vi "Live TDMS Viewer.vi"() -> ()   [LabVIEW 2019, in "Report Viewer.lvlib" / "Report Viewer.lvclass"]
doc: "Defer all the request for panel update the panel list. This will improve the loading time."
uses:
  Report Viewer.lvclass
  Custom Controls/Browse Tools.ctl
  <vilib>/Utility/tdmsutil.llb/fileViewerConfigData.ctl
panel:
  in  "tdms file in":refnum<k34>
  in  "Display Format":T1(ring)
  in  "Settings":bool
  in  "Properties / Values / Graph":T2(tab)=enum."Analog values (graph)"
  in  "Properties":i32(listbox)
  in  "Raw data values":i32(listbox)=-1
  out "Delta X (Time mS)":dbl
  out "Delta Y (Amplitude)":dbl
  out "Waveform Graph":waveform(dbl)[](graph)=[{"t0"=timestamp(0 s since 1904-01-01), "dt"=1.0, "Y"=[]}]
  in  "File contents":string[](tree)=["\"\u0000\u0000\u0000\u0002\u0000\u0000\u0000+Halt Mode Running_11:25:18.755 AM 11/6/2019\u0000\u0000\u0000\nPJB1_S CH0\""]
  in  "Open TDMS":bool
  in  "Save Graph":bool
  in  "Save Data":bool
  in  "Finished":bool
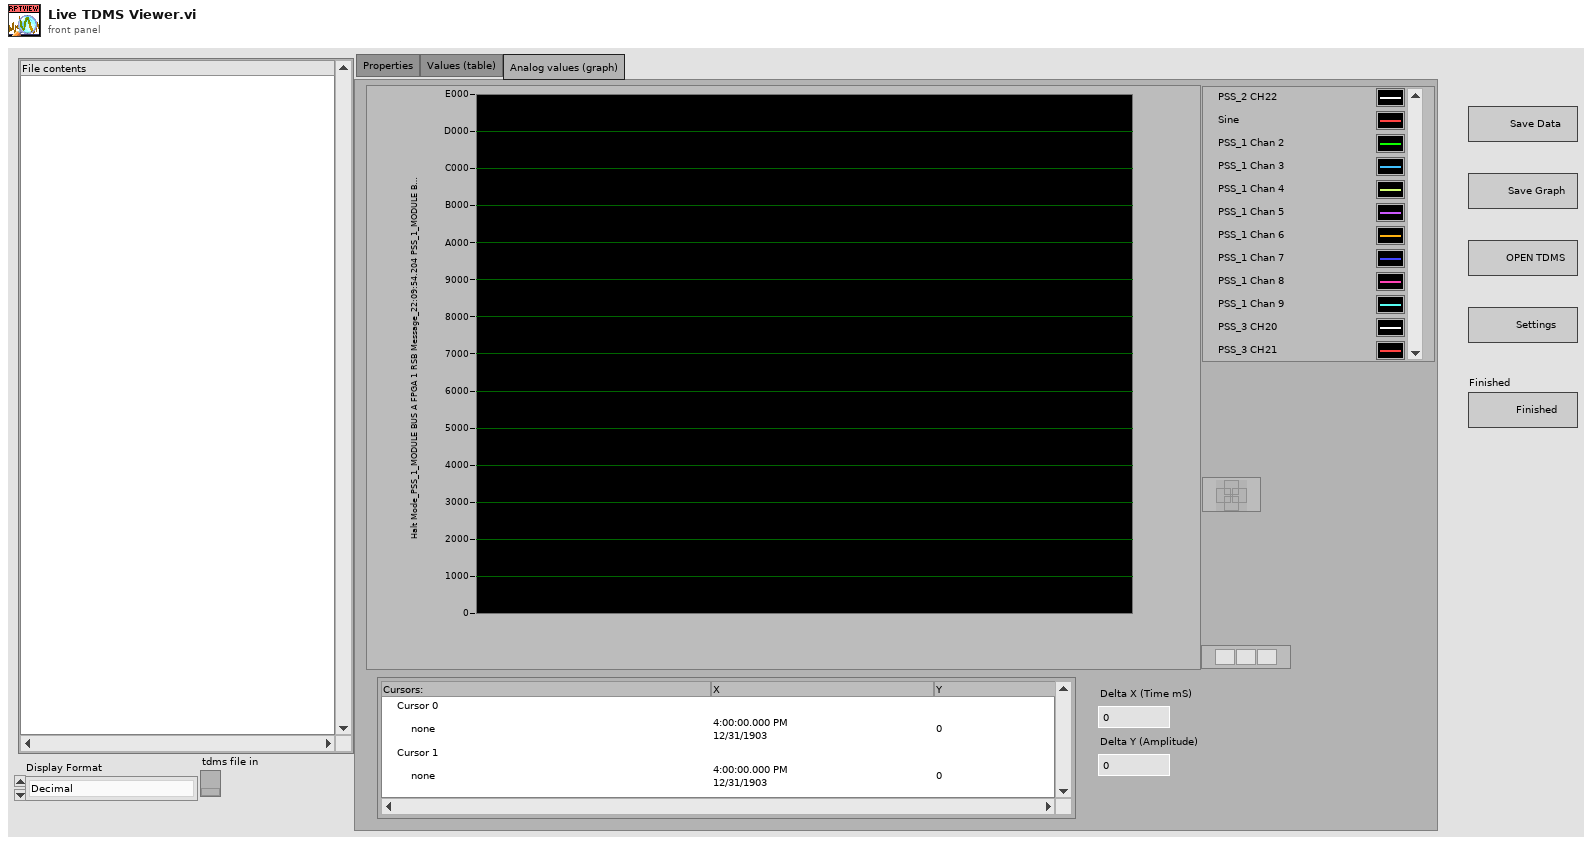
[diagram p1: front panel]
types:
  T1 = enum16{"Decimal", "Scientific", "Engineering", "Binary", "Octal", "Hexadecimal"}
  T2 = enum32{"Properties", "Values (table)", "Analog values (graph)"}
  T3 = typedef "fileViewerConfigData.ctl" = cluster{"Show all (table)":bool, "Show all (graph)":bool, "limit (table)":u64, "limit (graph)":u64, "no show":bool, "start (table)":u64, "start (graph)":u64}
  T4 = typedef "Report Viewer.lvlib/Report Viewer.lvclass/Browse Tools.ctl" = cluster{"Group":string, "Channel":string, "TDMS View Cfg":T3}
  T5 = typedef "imagedata.ctl" = cluster{"image type":i32, "image depth":i32, "image":u8[], "mask":u8[], "colors":u32[], "Rectangle":cluster{"left":i16, "top":i16, "right":i16, "bottom":i16}}
  T6 = typedef "LVCursorListTypeDef.ctl" = cluster{"Name":string, "Color":u32, "Style":u8, "Point Style":u8, "Name Visible":bool, "Allow Drag":bool, "Cursor Mode":u32, "Plot":i32, "Index":i32, "Position":cluster{"X":dbl, "Y":dbl}, "X Scale":u32, "Y Scale":u32, "Watch Plots":i32[], "Watch All Plots":bool, "Plot Area":i32, "Label Offset":cluster{"X":dbl, "Y":dbl}}[]
  T7 = cluster{"Name":string, "Color":u32, "Style":u8, "Point Style":u8, "Name Visible":bool, "Allow Drag":bool, "Cursor Mode":u32, "Plot":i32, "Index":i32, "Position":cluster{"X":dbl, "Y":dbl}, "X Scale":u32, "Y Scale":u32, "Watch Plots":i32[], "Watch All Plots":bool, "Plot Area":i32, "Label Offset":cluster{"X":dbl, "Y":dbl}}
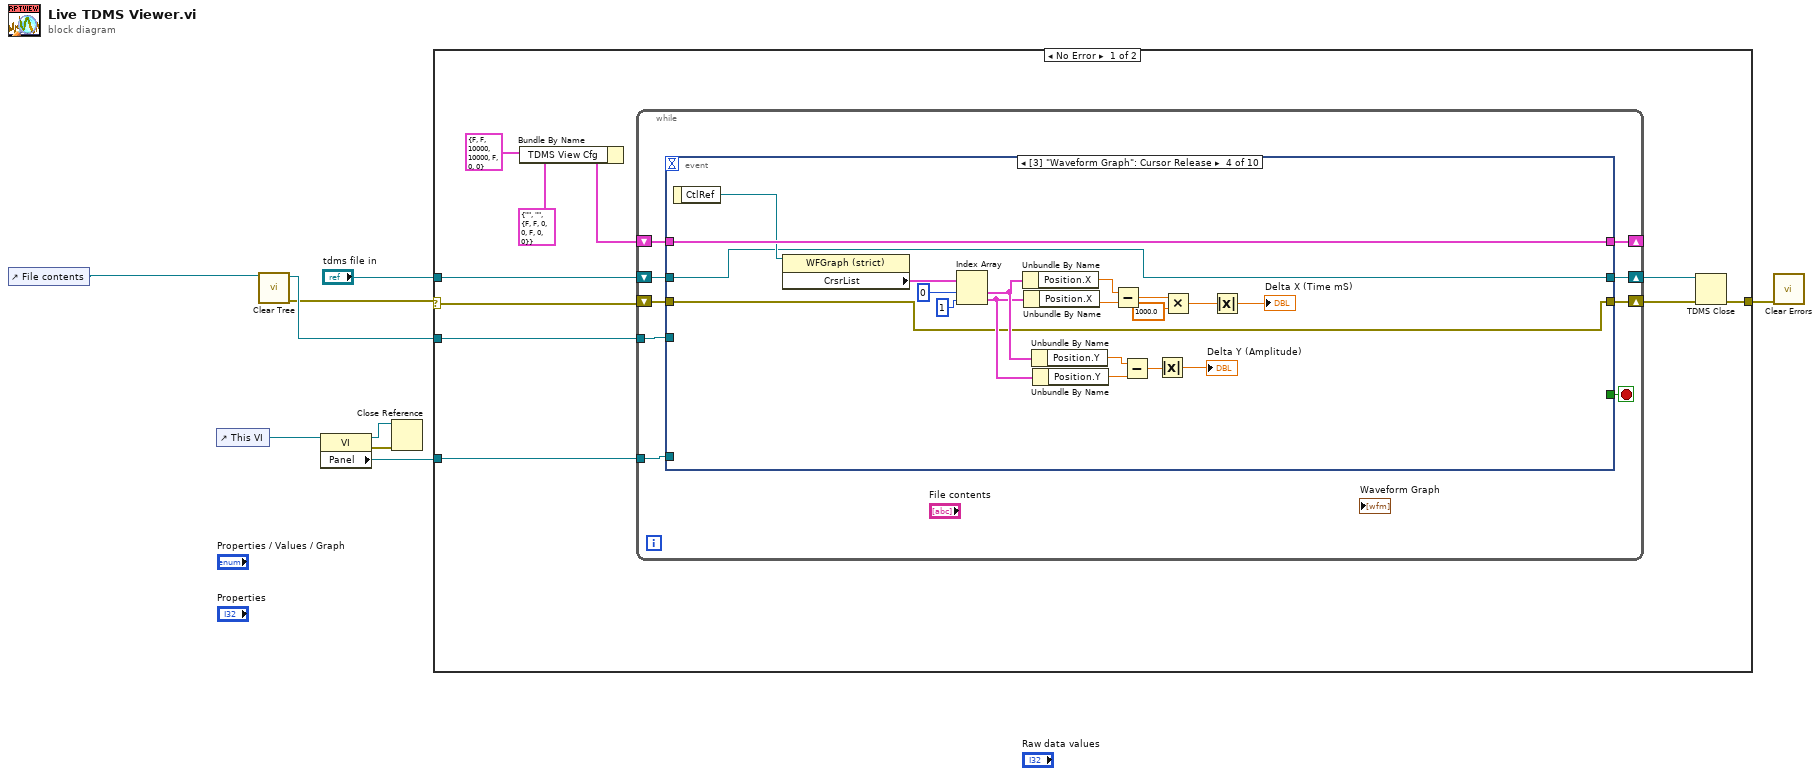
[diagram p0: block diagram]
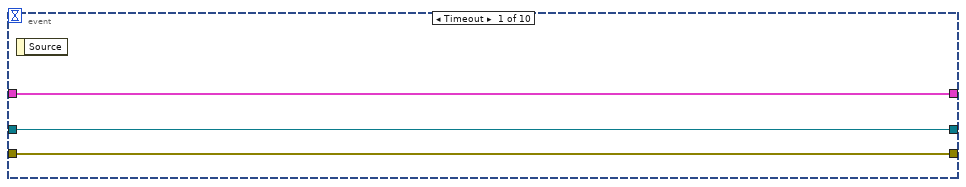
[diagram p2: hidden frame]
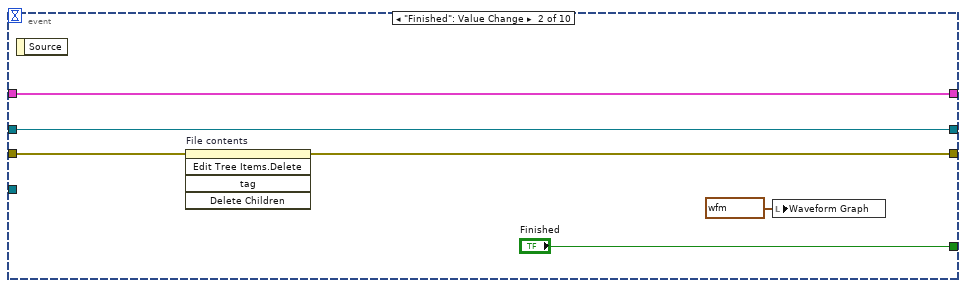
[diagram p3: hidden frame]
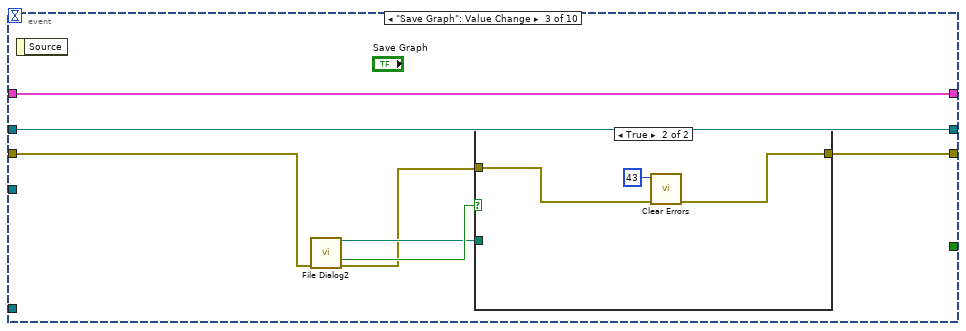
[diagram p4: hidden frame]
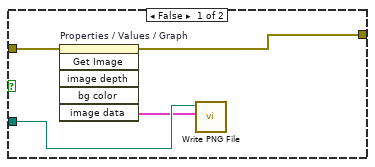
[diagram p5: hidden frame]
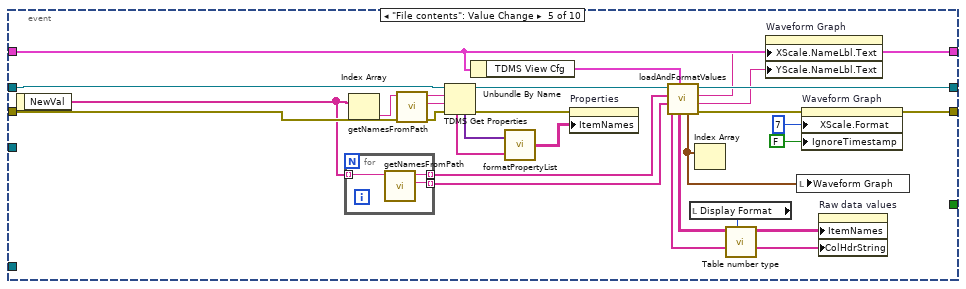
[diagram p6: hidden frame]
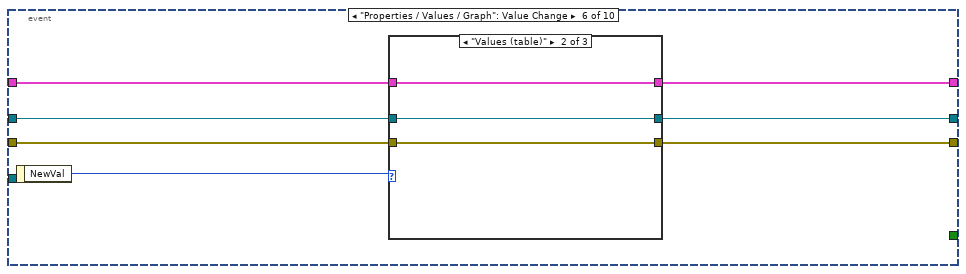
[diagram p7: hidden frame]
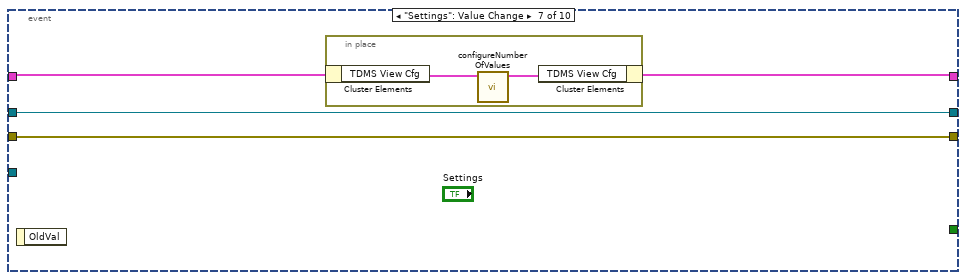
[diagram p10: hidden frame]
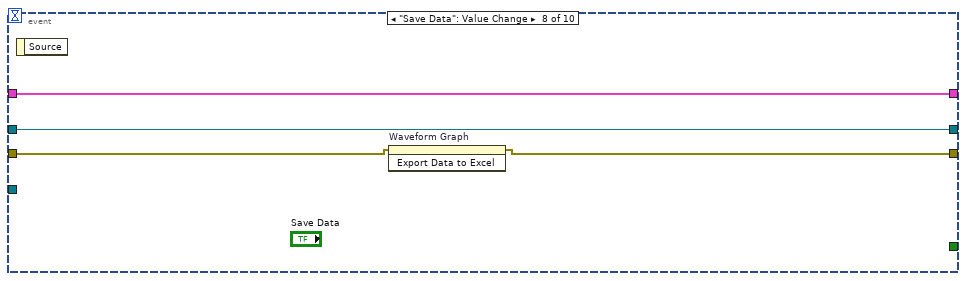
[diagram p11: hidden frame]
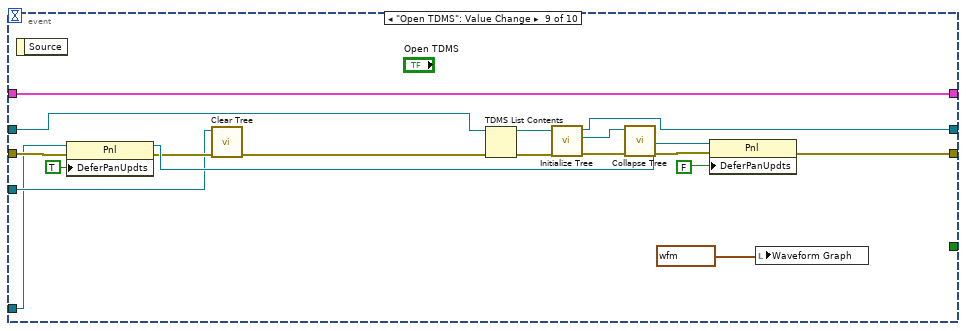
[diagram p12: hidden frame]
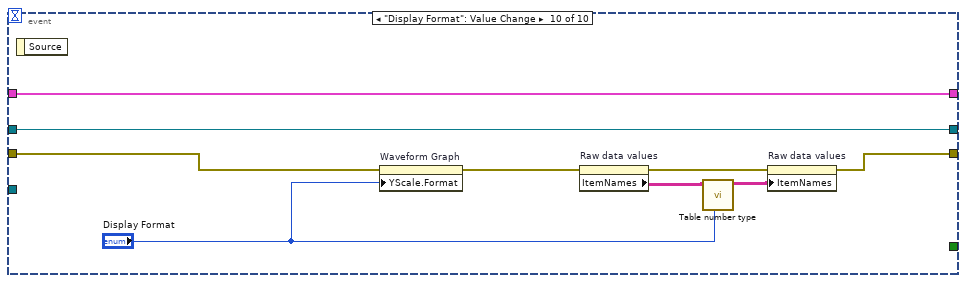
[diagram p13: hidden frame]
diagram:
  n1 = control-ref of="File contents"() -> (w1:refnum<vi>)
  n2 = control-ref of="This VI"() -> (w8:refnum<vi>)
  n3 = call "Clear Tree.vi"("reference"=w1) -> ("error out"=w4:errorcluster, "reference out"=w5:refnum<vi>)  [unwired: 9 in]
  n4 = property class="VI"(reference=w8) -> (reference out=w6:refnum<vi>, error out=w7:errorcluster, "Panel"=w3:refnum<vi>)  [unwired: 1 in]
  n5 = Close Reference(reference=w6, error in (no error)=w7) -> ()  [unwired: 1 out]
  n6 = case shown="No Error" w4 {
    selector: w4 -> [w12 w154]
    tunnel: [w19 w154] -> w9
    tunnel: w5 -> [w14 _]
    tunnel: w3 -> [w11 _]
    tunnel: "tdms file in" -> [w10 _]
    frame No Error {
      n7 = Bundle By Name(cluster=T4 {"Group"="", "Channel"="", "TDMS View Cfg"={"Show all (table)"=FALSE, "Show all (graph)"=FALSE, "limit (table)"=0, "limit (graph)"=0, "no show"=FALSE, "start (table)"=0, "start (graph)"=0}} ("Cluster"), "TDMS View Cfg"=T3 {"Show all (table)"=FALSE, "Show all (graph)"=FALSE, "limit (table)"=10000, "limit (graph)"=10000, "no show"=FALSE, "start (table)"=0, "start (graph)"=0} ("TDMS File Viewer Configuration")) -> (w16:T4)
      n8 = while {
        shift-right: [w26] -> w18
        shift-left: w12 -> [w27]
        shift-right: [w21] -> w13
        shift-left: w10 -> [w28]
        shift-right: [w23] -> _
        shift-left: w16 -> [w24]
        tunnel: w14 -> [w22]
        tunnel: w11 -> [w20]
        stop <- w25 stop-if-true
        n9 = event shown="[3] \"Waveform Graph\": Cursor Release" {
          selector: _ -> [_ _ _ _ _ _ _ _ _ _]
          dyn-events: _ -> [_ _ _ _ _ _ _ _ _ _]
          timeout: _ -> [_ _ _ _ _ _ _ _ _ _]
          tunnel: w28 -> [w29 w34 w41 w56 w75 w106 w117 w123 w128 w151]
          tunnel: w27 -> [w31 w32 w42 w55 w97 w102 w118 w125 w134 w152]
          tunnel: [w31 w32 w37 w55 w80 w101 w118 w124 w138 w149] -> w26
          tunnel: [_ "Finished" _ _ _ _ _ _ _ _] -> w25
          tunnel: w24 -> [w30 w35 w43 w69 w88 w105 w120 w126 w144 w153]
          tunnel: [w30 w35 w43 w69 w88 w104 w119 w126 w144 w153] -> w23
          tunnel: w22 -> [_ _ _ _ _ _ _ _ w131 _]
          tunnel: [w29 w34 w41 w56 w76 w103 w117 w123 w137 w151] -> w21
          tunnel: w20 -> [_ _ _ _ _ _ _ _ w130 _]
          event Timeout {
            n10 = event-data() -> ()  [unwired: 1 in, 1 out]
          }
          event "Finished": Value Change {
            n11 = event-data() -> ()  [unwired: 1 in, 1 out]
            n12 = invoke on="File contents" class="Tree (strict)" method="Edit Tree Items.Delete"(error in=w32) -> ()  [unwired: 4 in, 5 out]
            n13 = local write "Waveform Graph"(waveform(dbl)[] [{"t0"=timestamp(0 s since 1904-01-01), "dt"=1.0, "Y"=[]}] ("Waveform Graph")) -> ()
          }
          event "Save Graph": Value Change {
            n14 = event-data() -> ()  [unwired: 1 in, 1 out]
            n15 = call "File Dialog2"("error in"=w42) -> ("selected path"=w39:path, "cancelled"=w40:bool, "error out"=w38:errorcluster)  [unwired: 11 in, 1 out]
            n16 = case shown="True" w40 {
              tunnel: [w45 w48] -> w37
              tunnel: w38 -> [w46 w49]
              tunnel: w39 -> [w47 _]
              frame False {
                n17 = invoke on="Properties / Values / Graph" class="TabCtl (strict)" method="Get Image"(error in=w46) -> (error out=w45:errorcluster, "image data"=w44:T5)  [unwired: 5 in, 4 out]
                n18 = call <vilib>:"Write PNG File.vi"("image data"=w44, "path to PNG file"=w47) -> ()  [unwired: 8 in, 2 out]
              }
              frame True {
                n19 = call <vilib>:"Clear Errors.vi"("error in (no error)"=w49, "specific error code to clear (0: all)"=43) -> ("error out"=w48:errorcluster)  [unwired: 4 in, 1 out]
              }
            }
          }
          event "Waveform Graph": Cursor Release {
            n20 = event-data() -> ("CtlRef"=w57:refnum<vi>)  [unwired: 1 in]
            n21 = property on="Property Node" class="WFGraph (strict)"(reference=w57) -> ("CrsrList"=w68:T6)  [unwired: 1 in, 2 out]
            n22 = Index Array(array=w68, index #1=0 ("index"), index #2=1 ("index")) -> (element #1=w59:T7, element #2=w58:T7)
            n23 = Unbundle By Name(w59) -> ("Position.X"=w64:dbl)
            n24 = Unbundle By Name(w58) -> ("Position.X"=w65:dbl)
            n25 = Unbundle By Name(w59) -> ("Position.Y"=w60:dbl)
            n26 = Unbundle By Name(w58) -> ("Position.Y"=w61:dbl)
            n27 = Subtract(x=w64, y=w65) -> (x-y=w63:dbl)
            n28 = Subtract(x=w60, y=w61) -> (x-y=w52:dbl)
            n29 = Absolute Value(x=w52) -> (abs(x)=→"Delta Y (Amplitude)":dbl)
            n30 = Multiply(x=w63, y=1000.0) -> (x*y=w54:dbl)
            n31 = Absolute Value(x=w54) -> (abs(x)=→"Delta X (Time mS)":dbl)
          }
          event "File contents": Value Change {
            n32 = event-data() -> ("NewVal"=w85:string[])  [unwired: 1 in]
            n33 = for {
              tunnel: w85 -> [w100] mode=indexing
              tunnel: [w99] -> w84 mode=indexing
              tunnel: [w98] -> w83 mode=indexing
              n34 = call <vilib>:"getNamesFromPath.vi"("tree path"=w100) -> ("channel"=w98:string, "group"=w99:string)  [unwired: 1 in, 4 out]
            }
            n35 = Index Array(array=w85) -> (element=w89:string)  [unwired: 1 in]
            n36 = call <vilib>:"getNamesFromPath.vi"("error in (no error)"=w97, "tree path"=w89) -> ("error out"=w96:errorcluster, "channel"=w94:string, "group"=w95:string)  [unwired: 3 out]
            n37 = TDMS Get Properties(8:w96, 9:w94, 10:w95, 11:w75) -> (0:w90:errorcluster, 3:w86:refnum<k34>, 4:w93:variant[], 6:w92:string[])  [unwired: 4 out]
            n38 = Unbundle By Name(w88) -> ("TDMS View Cfg"=w87:T3)
            n39 = call <vilib>:"formatPropertyList.vi"("property names"=w92, "property values"=w93) -> ("strings"=w91:string[][])
            n40 = property on="Properties" class="MCListbox (strict)"(error in=w90, "ItemNames"=w91) -> ()  [unwired: 1 in, 2 out]
            n41 = call <vilib>:"loadAndFormatValues.vi"("configuration"=w87, "channel names"=w83, "group names"=w84, "tdms file"=w86) -> ("error out"=w81:errorcluster, "graph y names"=w73:string, "graph x names"=w74:string, "tdms file out"=w76:refnum<k34>, "waveform values"=w77:waveform(dbl)[], "table values"=w71:string[][], "table headers"=w82:string[])  [unwired: 1 in]
            n42 = local read "Display Format"() -> (w70:T1)
            n43 = Index Array(array=w77) -> ()  [unwired: 1 in, 1 out]
            n44 = call "Table number type.vi"("Y Scale.Display Format:Format"=w70, "Item Names in"=w71) -> ("Item Names out"=w72:string[][])  [unwired: 9 in]
            n45 = property on="Waveform Graph" class="WFGraph (strict)"("XScale.NameLbl.Text"=w74, "YScale.NameLbl.Text"=w73) -> ()  [unwired: 2 in, 2 out]
            n46 = local write "Waveform Graph"(w77) -> ()
            n47 = property on="Waveform Graph" class="WFGraph (strict)"(error in=w81, "XScale.Format"=u8 7 ("X Scale.Display Format:Format"), "IgnoreTimestamp"=FALSE ("Ignore Timestamp")) -> (error out=w80:errorcluster)  [unwired: 1 in, 1 out]
            n48 = property on="Raw data values" class="MCListbox (strict)"("ItemNames"=w72, "ColHdrString"=w82) -> ()  [unwired: 2 in, 2 out]
          }
          event "Properties / Values / Graph": Value Change {
            n49 = event-data() -> ("NewVal"=w107:T2)  [unwired: 1 in]
            n50 = case shown="\"Values (table)\"" w107 {
              tunnel: w106 -> [w110 w112 w115]
              tunnel: [w110 w112 w115] -> w103
              tunnel: w105 -> [w109 w113 w116]
              tunnel: [w109 w113 w116] -> w104
              tunnel: w102 -> [w108 w111 w114]
              tunnel: [w108 w111 w114] -> w101
              frame "Properties", Default {
              }
              frame "Values (table)" {
              }
              frame "Analog values (graph)" {
              }
            }
          }
          event "Settings": Value Change {
            n51 = event-data() -> ()  [unwired: 1 in, 1 out]
            n52 = in-place {
              n53 = in-place-cluster #1(w120) -> ("TDMS View Cfg"=w122:T3)
              n54 = call <vilib>:"configureNumberOfValues.vi"("TDMS File Viewer Configuration"=w122) -> ("TDMS File Viewer Configuration Out"=w121:T3)  [unwired: 10 out]
              n55 = in-place-cluster #1("TDMS View Cfg"=w121) -> (w119:T4)
            }
          }
          event "Save Data": Value Change {
            n56 = event-data() -> ()  [unwired: 1 in, 1 out]
            n57 = invoke on="Waveform Graph" class="WFGraph (strict)" method="Export Data to Excel"(error in=w125) -> (error out=w124:errorcluster)  [unwired: 2 in, 2 out]
          }
          event "Open TDMS": Value Change {
            n58 = event-data() -> ()  [unwired: 1 in, 1 out]
            n59 = property class="Pnl"(reference=w130, error in=w134, "DeferPanUpdts"=TRUE ("Defer Panel Updates")) -> (reference out=w133:refnum<vi>, error out=w132:errorcluster)
            n60 = call "Clear Tree.vi"("error in"=w132, "reference"=w131) -> ("error out"=w129:errorcluster)  [unwired: 8 in, 1 out]
            n61 = TDMS List Contents(4:w129, 7:w128) -> (0:w127:errorcluster, 3:w139:refnum<k34>)  [unwired: 1 in, 2 out]
            n62 = call "Initialize Tree.vi"("error in"=w127, "tdms file"=w139) -> ("error out"=w141:errorcluster, "tree reference out"=w142:refnum<vi>, "tdms file out"=w137:refnum<k34>)  [unwired: 7 in]
            n63 = call "Collapse Tree.vi"("error in (no error)"=w141, "Tree Ref in"=w142) -> ("error out"=w140:errorcluster)  [unwired: 8 in, 1 out]
            n64 = property class="Pnl"(reference=w133, error in=w140, "DeferPanUpdts"=FALSE ("Defer Panel Updates")) -> (error out=w138:errorcluster)  [unwired: 1 out]
            n65 = local write "Waveform Graph"(waveform(dbl)[] [{"t0"=timestamp(0 s since 1904-01-01), "dt"=1.0, "Y"=[]}] ("Waveform Graph")) -> ()
          }
          event "Display Format": Value Change {
            n66 = event-data() -> ()  [unwired: 1 in, 1 out]
            n67 = property on="Waveform Graph" class="WFGraph (strict)"(error in=w152, "YScale.Format"="Display Format") -> (error out=w150:errorcluster)  [unwired: 1 in, 1 out]
            n68 = property on="Raw data values" class="MCListbox (strict)"(error in=w150) -> (error out=w148:errorcluster, "ItemNames"=w147:string[][])  [unwired: 1 in, 1 out]
            n69 = call "Table number type.vi"("Y Scale.Display Format:Format"="Display Format", "Item Names in"=w147) -> ("Item Names out"=w146:string[][])  [unwired: 9 in]
            n70 = property on="Raw data values" class="MCListbox (strict)"(error in=w148, "ItemNames"=w146) -> (error out=w149:errorcluster)  [unwired: 1 in, 1 out]
          }
        }
      }
      n71 = TDMS Close(8:w18, 11:w13) -> (0:w19:errorcluster)  [unwired: 1 out]
    }
    frame Error {
    }
  }
  n72 = call <vilib>:"Clear Errors.vi"("error in (no error)"=w9) -> ()  [unwired: 5 in, 2 out]
